vi "Parse Log Entry.vi"(8 "error in":errorcluster, 11 "File name":path=path "C:/Data/April_2019/042419/sp0006_042419.tdms") -> (0 "error out":errorcluster, 2 "Lab notebook entry":string)   [LabVIEW 2024]
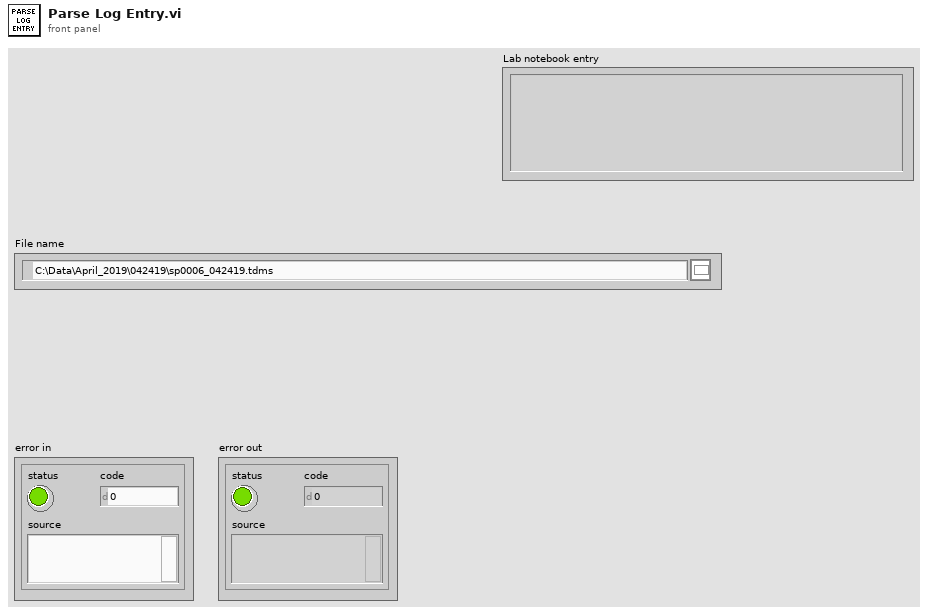
[diagram p1: front panel]
types:
  T1 = enum16{"open", "open or create", "create or replace", "create", "open (read-only)"}
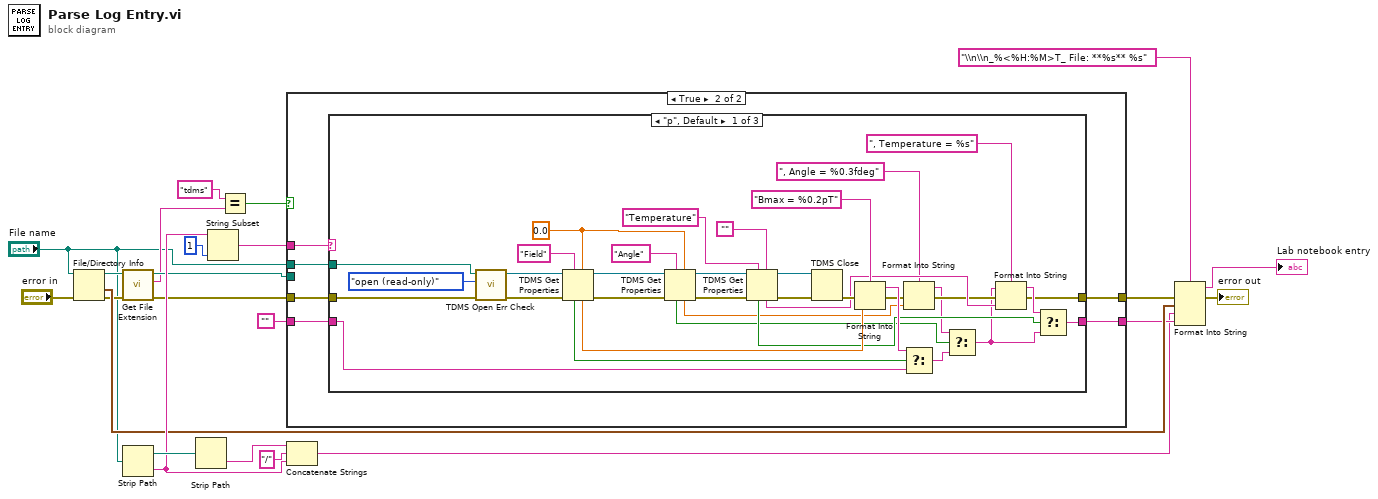
[diagram p0: block diagram]
diagram:
  n1 = File/Directory Info(path="File name", error in="error in") -> (path out=w16:path, last mod=w17:timestamp, error out=w15:errorcluster)  [unwired: 4 out]
  n2 = call <vilib>:"Get File Extension.vi"("error in (no error)"=w15, "file"=w16) -> ("error out"=w14:errorcluster, "lowercase file extension"=w11:string, "dup file"=w13:path)  [unwired: 5 in, 2 out]
  n3 = Strip Path(path="File name") -> (stripped path=w23:path, name=w18:string)
  n4 = Strip Path(path=w23) -> (name=w2:string)  [unwired: 1 out]
  n5 = String Subset(string=w18, length (rest)=1 ("length (rest)")) -> (substring=w8:string)  [unwired: 1 in]
  n6 = Equal?(x="tdms", y=w11) -> (x = y?=w10:bool)
  n7 = case shown="True" w10 {
    tunnel: w14 -> [w25 w26]
    tunnel: w13 -> [_ _]
    tunnel: w8 -> [_ w31]
    tunnel: "File name" -> [_ w30]
    tunnel: "" -> [w24 w29]
    tunnel: [w24 w28] -> w5
    tunnel: [w25 w27] -> w4
    frame False {
    }
    frame True {
      n8 = case shown="\"p\", Default" w31 {
        tunnel: [w46 w68 _] -> w28
        tunnel: w30 -> [w67 _ _]
        tunnel: w26 -> [w65 w69 w70]
        tunnel: [w47 w69 w70] -> w27
        tunnel: w29 -> [w56 w68 _]
        frame "p", Default {
          w41 = 0.0
          n9 = call "TDMS Open Err Check.vi"("Error In"=w65, "operation (0:open)"=T1."open (read-only)", "File Path Control"=w67) -> ("Error Out"=w63:errorcluster, "tdms file out"=w64:refnum<k34>)  [unwired: 6 in, 1 out]
          n10 = TDMS Get Properties(5:w41, 7:"Field" ("property name"), 8:w63, 11:w64) -> (0:w45:errorcluster, 3:w43:refnum<k34>, 4:w59:dbl, 6:w61:bool)  [unwired: 2 in, 2 out]
          n11 = TDMS Get Properties(5:w41, 7:"Angle" ("property name"), 8:w45, 11:w43) -> (0:w44:errorcluster, 3:w42:refnum<k34>, 4:w36:dbl, 6:w32:bool)  [unwired: 2 in, 2 out]
          n12 = TDMS Get Properties(5:"", 7:"Temperature" ("property name"), 8:w44, 11:w42) -> (0:w55:errorcluster, 3:w54:refnum<k34>, 4:w48:string, 6:w51:bool)  [unwired: 2 in, 2 out]
          n13 = TDMS Close(8:w55, 11:w54) -> (0:w60:errorcluster)  [unwired: 1 out]
          n14 = Format Into String(format string="Bmax = %0.2pT" ("Rendered metadata"), error in=w60, w59) -> (resulting string=w57:string, error out=w39:errorcluster)  [unwired: 1 in]
          n15 = Format Into String(format string=", Angle = %0.3fdeg" ("Rendered metadata"), error in=w39, w36) -> (resulting string=w34:string, error out=w38:errorcluster)  [unwired: 1 in]
          n16 = Select(t=w57, s=w61, f=w56) -> (s? t:f=w33:string)
          n17 = Select(t=w34, s=w32, f=w33) -> (s? t:f=w35:string)
          n18 = Format Into String(format string=", Temperature = %s" ("Rendered metadata"), initial string=w35, error in=w38, w48) -> (resulting string=w50:string, error out=w47:errorcluster)
          n19 = Select(t=w50, s=w51, f=w35) -> (s? t:f=w46:string)
        }
        frame "m" {
        }
        frame "s" {
        }
      }
    }
  }
  n20 = Concatenate Strings(w2, "/" ("string"), w18) -> (w3:string)
  n21 = Format Into String(format string="\\n\\n_%<%H:%M>T_ File: **%s** %s", error in=w4, w17, w3, w5) -> (resulting string=→"Lab notebook entry":string, error out=→"error out":errorcluster)  [unwired: 1 in]
